vi "Get Object Entry Count.vi"(8 "error in":errorcluster, 11 "Obj Dict in":refnum<class "Object Dictionary.lvclass">) -> (0 "error out":errorcluster, 2 "Count":i32, 3 "Obj Dict out":refnum<class "Object Dictionary.lvclass">)   [LabVIEW 2020, in "CANopen.lvlib" / "Object Dictionary.lvclass"]
uses:
  Object Dictionary.lvclass
  Object Dictionary.lvclass/Object Dictionary.ctl
  Ordered-Dictionary/Ordered Object Dictionary/Source/Ordered Object Dictionary.lvclass/Ordered Object Dictionary.ctl
  Ordered-Dictionary/Ordered Object Dictionary/Source/Ordered Object Dictionary.lvclass
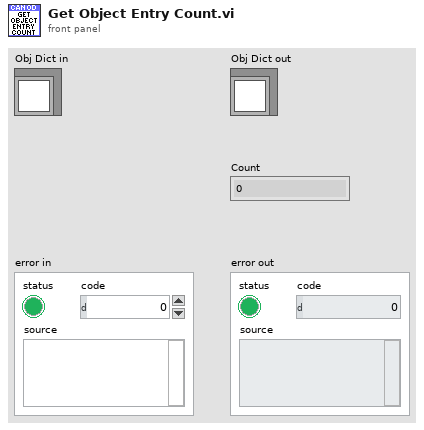
[diagram p1: front panel]
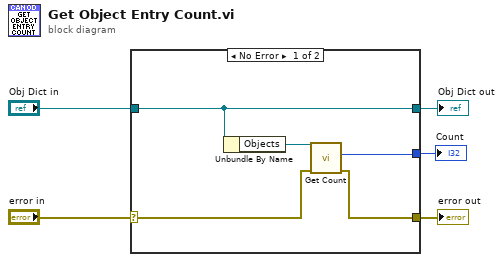
[diagram p0: block diagram]
diagram:
  n1 = case shown="No Error" "error in" {
    selector: "error in" -> [w8 w12]
    tunnel: [w7 w12] -> w2
    tunnel: [w10 w11] -> w4
    tunnel: "Obj Dict in" -> [w10 w11]
    tunnel: [w6 _] -> w1
    frame No Error {
      n2 = Unbundle By Name(w10) -> ("Objects"=w9:refnum<class "Ordered Object Dictionary.lvclass">)
      n3 = call "Get Count.vi"("error in"=w8, "Ordered Object Dictionary in"=w9) -> ("error out"=w7:errorcluster, "Count"=w6:i32)  [unwired: 7 in, 1 out]
    }
    frame Error {
    }
  }
  "Obj Dict out" <- w4
  "error out" <- w2
  "Count" <- w1
